vi "Main NR.vi"(8 "error in":errorcluster, 11 "FPGA Read in":refnum<class "FPGA Read.lvclass">) -> (0 "error out":errorcluster, 3 "FPGA Read out":refnum<class "FPGA Read.lvclass">)   [LabVIEW 2017, in "FPGA Read.lvclass"]
doc: "The <b>Queued Message Handler</b> of the Worker that owns this VI."
uses:
  FPGA Read.lvclass
  Initialization Data.ctl
  Response Cases.ctl
  <vilib>/addons/_Workers/Library/Case Label.ctl
  FPGA Read.lvclass/FPGA Read.ctl
  rsp_Receive FPGA Data.ctl
  rqp_Start FPGA.ctl
  <vilib>/LabVIEW Targets/FPGA/cRIO/shared/nicrio_ModuleControls/nicrio_cRIO-9205_VoltageRange.ctl
  <vilib>/LabVIEW Targets/FPGA/cRIO/shared/nicrio_ModuleControls/nicrio_cRIO-9205_TerminalMode.ctl
  <vilib>/FPGAPlugInAG/Dynamic/niLvFpga_Close_Dynamic.vi
  <vilib>/Utility/error.llb/Error Cluster From Error Code.vi
  <vilib>/rvi/errors/niLvFpgaAdjustHostInterfaceError.vi
  <vilib>/FPGAPlugInAG/cRIO-9067/niLvFpga_Open_cRIO-9067.vi
  <vilib>/rvi/interface/common/dynamic/niFpgaDynamicAddResources.vi
  <vilib>/FPGAPlugInAG/Dynamic/niLvFpga_Run_Dynamic.vi
  <vilib>/rvi/interface/nirviCloseFPGA/nirviCloseFPGA.xnode
  FPGA Reference.ctl
  <vilib>/rvi/interface/nirviMethod/nirviMethod.xnode
  <vilib>/rvi/interface/nirviOpenFPGA/nirviOpenFPGA.xnode
  FPGA Bitfiles/cRIONI9205Demo_FPGATarget_FPGAMain_SCyGEa71Jm4.lvbitx
  FPGA Main.vi
  <vilib>/rvi/interface/nirviReadWriteControl/nirviReadWriteControl.xnode
  <vilib>/FPGAPlugInAG/Dynamic/niLvFpga_ReadFifo_Dynamic.vi
  <vilib>/rvi/errors/niLvFpgaMergeErrorWithErrorCode.vi
  NiFpgaLv.dll
  <vilib>/rvi/interface/Simulation/niFpgaSimulationCallBeginRW.vi
  <vilib>/addons/_Workers/Library/Workers.lvlib
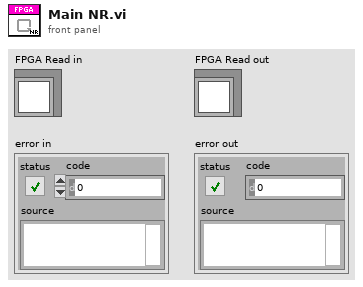
[diagram p1: front panel]
types:
  T1 = typedef "FPGA Read.lvclass/Initialization Data.ctl" = cluster{"Response Cases":T2}
  T2 = typedef "FPGA Read.lvclass/Response Cases.ctl" = cluster{"Receive FPGA Data":T3}
  T3 = typedef "Workers.lvlib/Case Label.ctl" = string
  T4 = typedef "FPGA Read.lvclass/rsp_Receive FPGA Data.ctl" = cluster{"FPGA Data":fxp<+/-,26,5>[]}
  T5 = typedef "nicrio_cRIO-9205_VoltageRange.ctl" = enum8{"+/- 10V", "+/- 5V", "+/- 1V", "+/- 200mV"}
  T6 = typedef "nicrio_cRIO-9205_TerminalMode.ctl" = enum8{"RSE", "NRSE", "DIFF"}
  T7 = cluster{"Voltage Range":T5, "Terminal Mode":T6}[]
  T8 = typedef "FPGA Read.lvclass/rqp_Start FPGA.ctl" = cluster{"String":string}
  T9 = typedef "FPGA Read.lvclass/FPGA Reference.ctl" = refnum<k20>
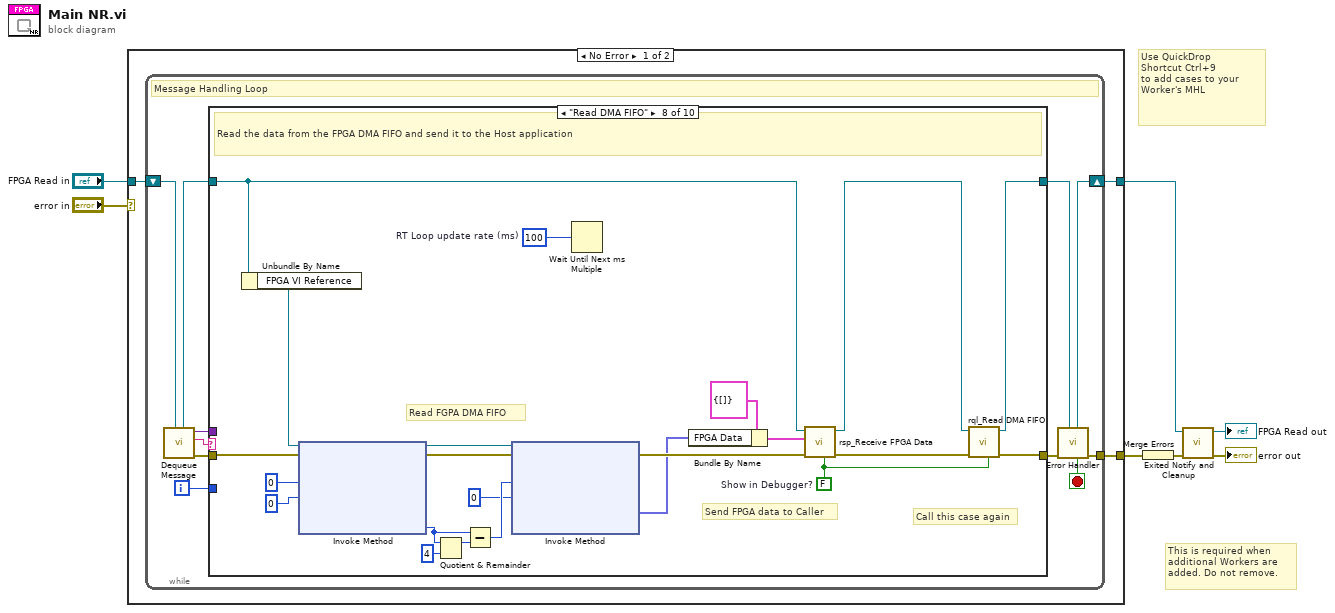
[diagram p0: block diagram]
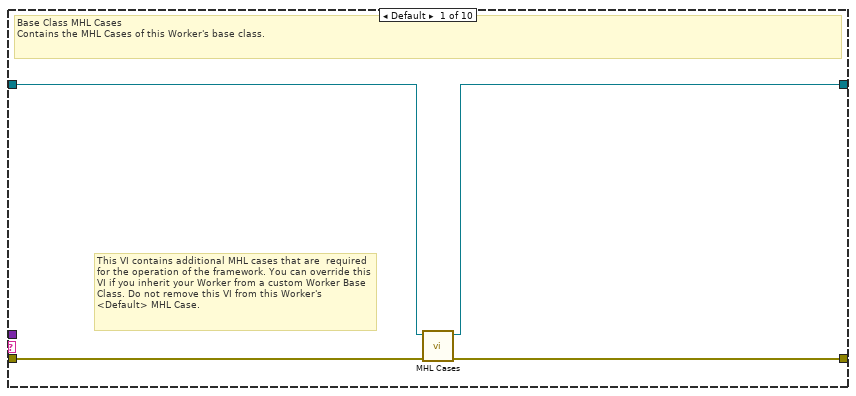
[diagram p2: hidden frame]
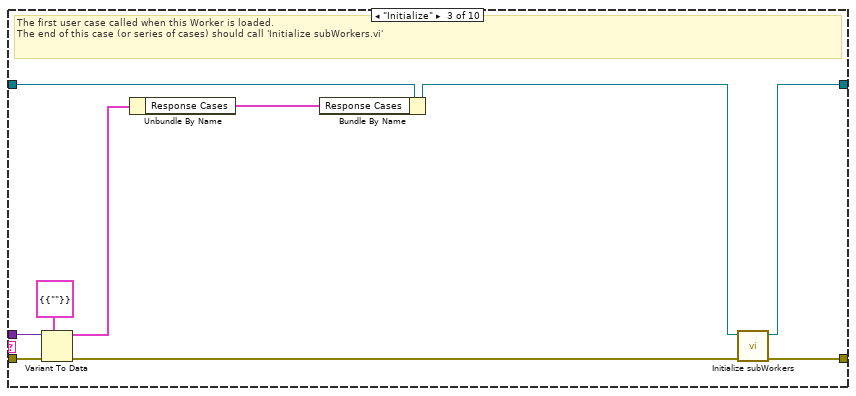
[diagram p4: hidden frame]
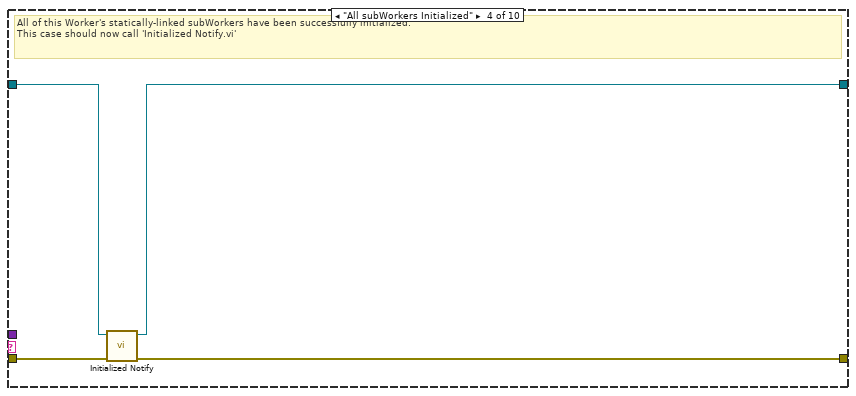
[diagram p5: hidden frame]
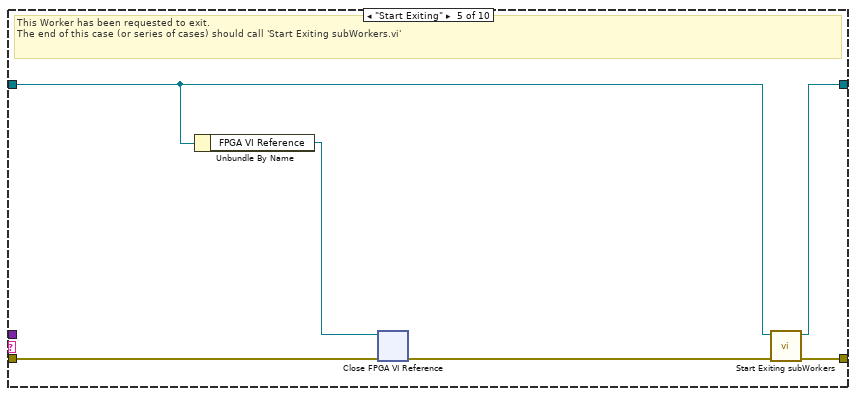
[diagram p6: hidden frame]
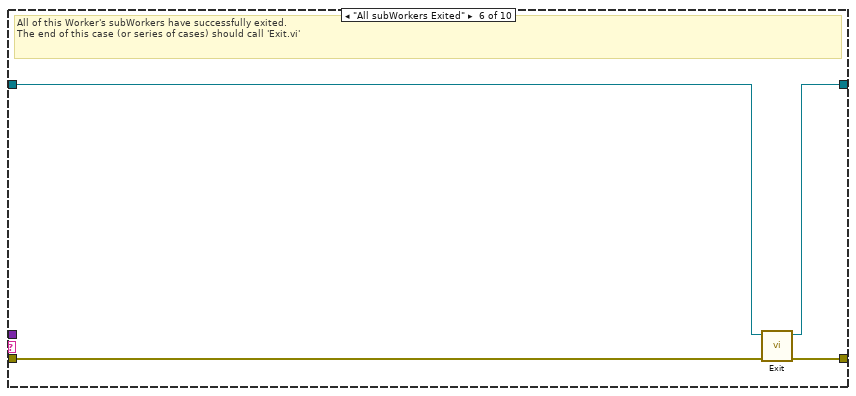
[diagram p7: hidden frame]
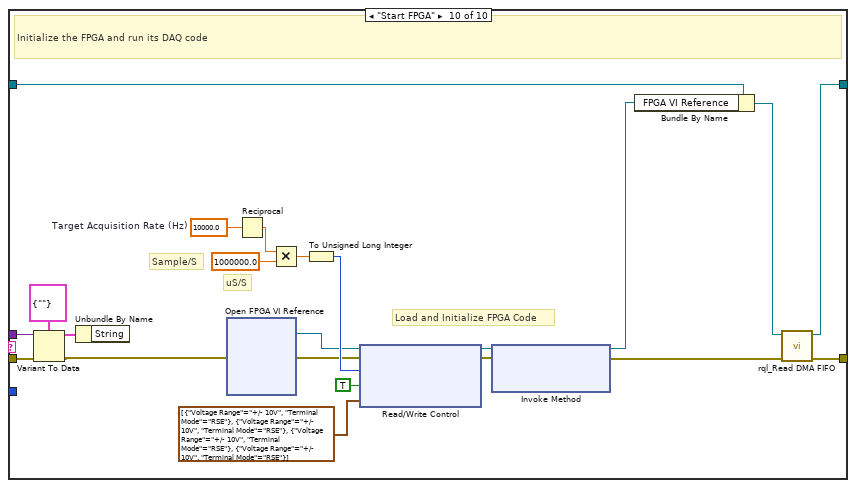
[diagram p10: hidden frame]
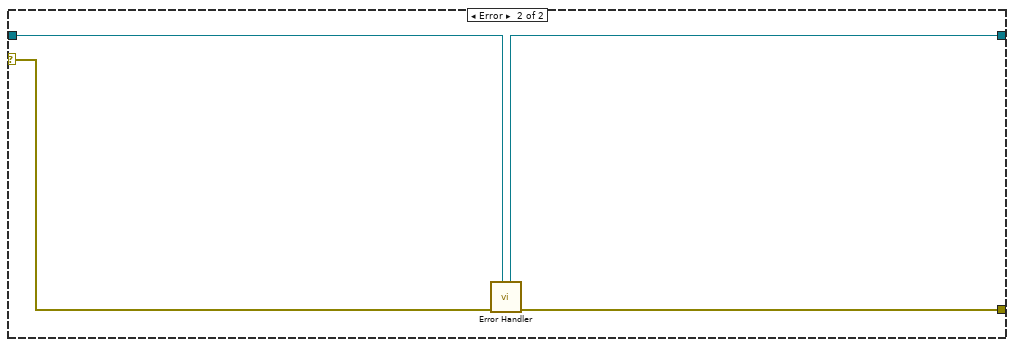
[diagram p11: hidden frame]
diagram:
  # "Use QuickDrop\nShortcut Ctrl+9\nto add cases to your\nWorker's MHL"
  # "This is required when additional Workers are added. Do not remove."
  n1 = case shown="No Error" "error in" {
    tunnel: "FPGA Read in" -> [w8 w101]
    tunnel: [w10 w102] -> w6
    tunnel: [w9 w100] -> w7
    selector: "error in" -> [_ w103]
    frame No Error {
      n2 = while {
        shift-right: [w19] -> w9
        shift-left: w8 -> [w21]
        tunnel: [w20] -> w10
        i -> [w12]
        stop <- w13 stop-if-true
        # "Message Handling Loop"
        n3 = call-dynamic "Dequeue Message.vi"("Worker"=w21) -> ("error out"=w18:errorcluster, "Case out"=w14:string, "Data out"=w11:variant, "Worker out"=w16:refnum<class "FPGA Read.lvclass">)  [unwired: 6 in, 1 out]
        n4 = case "Worker MHL Case Structure (DO NOT CHANGE LABEL NAME)" shown="\"Read DMA FIFO\"" w14 {
          tunnel: w18 -> [w25 w26 w35 w41 w45 w51 w53 w65 w77 w99]
          tunnel: [w24 w26 w37 w40 w47 w50 w53 w63 w77 w79] -> w17
          tunnel: w16 -> [w23 w27 w30 w39 w43 w49 w52 w59 w76 w81]
          tunnel: [w22 w27 w36 w38 w46 w48 w52 w62 w76 w80] -> w15
          tunnel: w12 -> [_ _ _ _ _ _ _ _ _ _]
          tunnel: w11 -> [_ _ w33 _ _ _ _ _ _ w97]
          frame Default {
            # "This VI contains additional MHL cases that are  required for the operation of the framework. You can override this VI if you inherit your Worker from a custom Worker Base Class. Do not remove this VI from this Worker's <Default> MHL Case."
            # "Base Class MHL Cases\nContains the MHL Cases of this Worker's base class."
            n5 = call-dynamic "MHL Cases.vi"("error in"=w25, "Worker in"=w23) -> ("error out"=w24:errorcluster, "Worker out"=w22:refnum<class "FPGA Read.lvclass">)  [unwired: 8 in]
          }
          frame "------------ FRAMEWORK CASES -----------" {
            # "Start of Workers Framework Cases"
          }
          frame "Initialize" {
            # "The first user case called when this Worker is loaded.\nThe end of this case (or series of cases) should call 'Initialize subWorkers.vi'"
            n6 = Variant To Data(error in=w35, type=T1 {"Response Cases"={"Receive FPGA Data"=""}} ("Cluster"), Variant=w33) -> (data=w31:T1, error out=w34:errorcluster)
            n7 = Unbundle By Name(w31) -> ("Response Cases"=w32:T2)
            n8 = Bundle By Name(cluster=w30, "Response Cases"=w32) -> (w29:refnum<class "FPGA Read.lvclass">)
            n9 = call-dynamic "Initialize subWorkers.vi"("error in"=w34, "Worker"=w29) -> ("error out"=w37:errorcluster, "dup Worker out"=w36:refnum<class "FPGA Read.lvclass">)  [unwired: 8 in]
          }
          frame "All subWorkers Initialized" {
            # "All of this Worker's statically-linked subWorkers have been successfully initialized.\nThis case should now call 'Initialized Notify.vi'"
            n10 = call-dynamic "Initialized Notify.vi"("error in"=w41, "Worker"=w39) -> ("error out"=w40:errorcluster, "dup Worker out"=w38:refnum<class "FPGA Read.lvclass">)  [unwired: 8 in]
          }
          frame "Start Exiting" {
            # "This Worker has been requested to exit. \nThe end of this case (or series of cases) should call 'Start Exiting subWorkers.vi'"
            n11 = Unbundle By Name(w43) -> ("FPGA VI Reference"=w42:T9)
            n12 = xnode "Close FPGA VI Reference"("FPGA VI Reference In"=w42, "error in"=w45) -> ("error out"=w44:errorcluster)
            n13 = call-dynamic "Start Exiting subWorkers.vi"("error_in"=w44, "Worker"=w43) -> ("error out"=w47:errorcluster, "dup Worker out"=w46:refnum<class "FPGA Read.lvclass">)  [unwired: 8 in]
          }
          frame "All subWorkers Exited" {
            # "All of this Worker's subWorkers have successfully exited. \nThe end of this case (or series of cases) should call 'Exit.vi'"
            n14 = call-dynamic "Exit.vi"("error_in"=w51, "Worker"=w49) -> ("error out"=w50:errorcluster, "dup Worker out"=w48:refnum<class "FPGA Read.lvclass">)  [unwired: 8 in]
          }
          frame "------------- LOCAL API CASES -------------" {
            # "Start of Workers Local API Cases"
          }
          frame "Read DMA FIFO" {
            w54 = FALSE  # Show in Debugger?
            w75 = u32 100  # RT Loop update rate (ms)
            # "Read FGPA DMA FIFO"
            # "Call this case again"
            # "Send FPGA data to Caller"
            # "Read the data from the FPGA DMA FIFO and send it to the Host application"
            n15 = Unbundle By Name(w59) -> ("FPGA VI Reference"=w64:T9)
            n16 = xnode "Invoke Method"("FPGA VI Reference In"=w64, "error in"=w65, "Number of Elements"=u32 0, "Timeout (ms)"=0) -> ("FPGA VI Reference Out"=w72:T9, "error out"=w66:errorcluster, "Elements Remaining"=w69:u32)  [unwired: 1 out]
            n17 = Quotient & Remainder(x=w69, y=u32 4) -> (x-y*floor(x/y)=w70:u32)  [unwired: 1 out]
            n18 = Subtract(x=w69, y=w70) -> (x-y=w68:u32)
            n19 = xnode "Invoke Method"("FPGA VI Reference In"=w72, "error in"=w66, "Number of Elements"=w68, "Timeout (ms)"=0) -> ("error out"=w61:errorcluster, "Data"=w55:fxp<+/-,26,5>[])  [unwired: 2 out]
            n20 = Wait Until Next ms Multiple(millisecond multiple=w75) -> ()  [unwired: 1 out]
            n21 = Bundle By Name(cluster=T4 {"FPGA Data"=[]} ("Data in"), "FPGA Data"=w55) -> (w56:T4)
            n22 = call "rsp_Receive FPGA Data.vi"("Show in Debugger?"=w54, "error in"=w61, "Data in"=w56, "FPGA Read in"=w59) -> ("error out"=w60:errorcluster, "dup FPGA Read out"=w58:refnum<class "FPGA Read.lvclass">)  [unwired: 6 in]
            n23 = call "rql_Read DMA FIFO.vi"("Show in Debugger?"=w54, "error in"=w60, "FPGA Read in"=w58) -> ("error out"=w63:errorcluster, "dup FPGA Read out"=w62:refnum<class "FPGA Read.lvclass">)  [unwired: 7 in]
          }
          frame "------------- PUBLIC API CASES -------------" {
            # "Start of Workers Public API Cases"
          }
          frame "Start FPGA" {
            w88 = 10000.0  # Target Acquisition Rate (Hz)
            # "Load and Initialize FPGA Code"
            # "Sample/S"
            # "uS/S"
            # "Initialize the FPGA and run its DAQ code"
            n24 = Variant To Data(error in=w99, type=T8 {"String"=""} ("Data"), Variant=w97) -> (data=w96:T8, error out=w78:errorcluster)
            n25 = Unbundle By Name(w96) -> ()  [unwired: 1 out]
            n26 = xnode "Open FPGA VI Reference"("error in"=w78) -> ("FPGA VI Reference Out"=w85:refnum<k20>, "error out"=w86:errorcluster)  [unwired: 1 in]
            n27 = Reciprocal(x=w88) -> (1/x=w89:dbl)
            n28 = Multiply(x=w89, y=1000000.0) -> (x*y=w91:dbl)
            n29 = To Unsigned Long Integer(number=w91) -> (unsigned 32bit integer=w92:u32)
            n30 = xnode "Read/Write Control"("FPGA VI Reference In"=w85, "error in"=w86, "Loop Rate (uS)"=w92, "Update AI Settings"=TRUE, "AI Channel Settings"=T7 [{"Voltage Range"=enum."+/- 10V", "Terminal Mode"=enum."RSE"}, {"Voltage Range"=enum."+/- 10V", "Terminal Mode"=enum."RSE"}, {"Voltage Range"=enum."+/- 10V", "Terminal Mode"=enum."RSE"}, {"Voltage Range"=enum."+/- 10V", "Terminal Mode"=enum."RSE"}]) -> ("FPGA VI Reference Out"=w93:refnum<k20>, "error out"=w94:errorcluster)
            n31 = xnode "Invoke Method"("FPGA VI Reference In"=w93, "error in"=w94) -> ("FPGA VI Reference Out"=w83:refnum<k20>, "error out"=w84:errorcluster)  [unwired: 1 in]
            n32 = Bundle By Name(cluster=w81, "FPGA VI Reference"=w83) -> (w82:refnum<class "FPGA Read.lvclass">)
            n33 = call "rql_Read DMA FIFO.vi"("error in"=w84, "FPGA Read in"=w82) -> ("error out"=w79:errorcluster, "dup FPGA Read out"=w80:refnum<class "FPGA Read.lvclass">)  [unwired: 8 in]
          }
        }
        n34 = call-dynamic "Error Handler.vi"("Worker"=w15, "error_in"=w17) -> ("error out"=w20:errorcluster, "Stop Loop"=w13:bool, "Worker out"=w19:refnum<class "FPGA Read.lvclass">)  [unwired: 7 in]
      }
    }
    frame Error {
      n35 = call-dynamic "Error Handler.vi"("Worker"=w101, "error_in"=w103) -> ("error out"=w102:errorcluster, "Worker out"=w100:refnum<class "FPGA Read.lvclass">)  [unwired: 7 in, 1 out]
    }
  }
  n36 = Merge Errors(w6) -> (w3:errorcluster)
  n37 = call-dynamic "Exited Notify and Cleanup.vi"("error_in"=w3, "Worker"=w7) -> ("error out"=→"error out":errorcluster, "dup Worker out"=→"FPGA Read out":refnum<class "FPGA Read.lvclass">)  [unwired: 8 in]
